vi "Get Exp Time.vi"(0 "Notifier Name":string, 11 "Error In":errorcluster) -> (4 "Notifier Name DUP":string, 8 "Exp Time (s)":dbl, 15 "Error Out":errorcluster)   [LabVIEW 2020]
uses:
  Hardware Configuration/Hardware Configuration Controls/Company.ctl
  Hamamatsu/Orca Flash/Orca Flash Controls/Orca Flash Parameters.ctl
  Hamamatsu/Orca Flash/Orca Flash Controls/Orca Flash Parameter List.ctl
  Hamamatsu/Orca Flash/Orca Flash Controls/Orca Flash Actions.ctl
  IDS/IDS Controls/IDS Actions.ctl
  IDS/IDS Controls/IDS Parameters.ctl
  IDS/IDS Controls/IDS Parameter List.ctl
  Photometrics/Prime BSI/R Cubed SITK/Prime BSI R3 Controls/Prime R3 Actions.ctl
  Photometrics/Prime BSI/R Cubed SITK/Prime BSI R3 Controls/Prime R3 Parameters.ctl
  Photometrics/Prime BSI/R Cubed SITK/Prime BSI R3 Controls/Prime R3 Parameter List.ctl
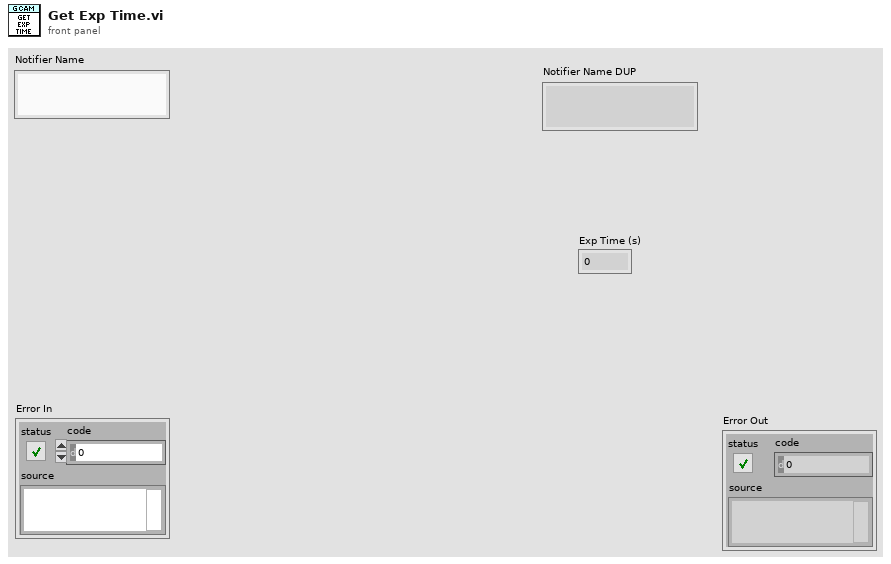
[diagram p1: front panel]
types:
  T1 = typedef "Company.ctl" = enum16{"AA Opto Electronic", "ASI", "Coherent", "Creset Optics", "CVI", "DAQmx", "Hamamatsu", "IDS", "Mad City Labs", "Marzhauser", "Measurement Computing", "MPB Com", "Olympus", "Photometrics", "PI", "Prior", "Thorlabs"}
  T2 = typedef "Orca Flash Actions.ctl" = enum16{"Idle", "Preview", "Record", "Record Settings", "Set Param", "Get Param", "Set ROI", "Get ROI", "Trigger Source", "Trigger Type", "Progessive Mode", "Area Mode", "Status", "Quit"}
  T3 = typedef "Orca Flash Parameters.ctl" = cluster{"Value":dbl, "Parameter":T4}
  T4 = typedef "Orca Flash Parameter List.ctl" = u32
  T5 = typedef "IDS Parameter List.ctl" = enum16{"Exposure Time (s)", "Binning"}
  T6 = typedef "IDS Parameters.ctl" = cluster{"Parameter":T5, "Value":dbl}
  T7 = typedef "IDS Actions.ctl" = enum16{"Error Check", "Initialize", "Preview", "Record", "Abort", "Record Settings", "Set Parameter", "Get Parameter", "Set ROI", "Get ROI", "Status", "Quit"}
  T8 = typedef "Prime R3 Parameter List.ctl" = enum16{"Exposure Time (s)"}
  T9 = typedef "Prime R3 Parameters.ctl" = cluster{"Parameter":T8, "Value":dbl}
  T10 = typedef "Prime R3 Actions.ctl" = enum16{"Error Check", "Initialize", "Preview", "Record", "Abort", "Record Settings", "Set Parameter", "Get Parameter", "Set ROI", "Get ROI", "Status", "Set Trigger", "Quit"}
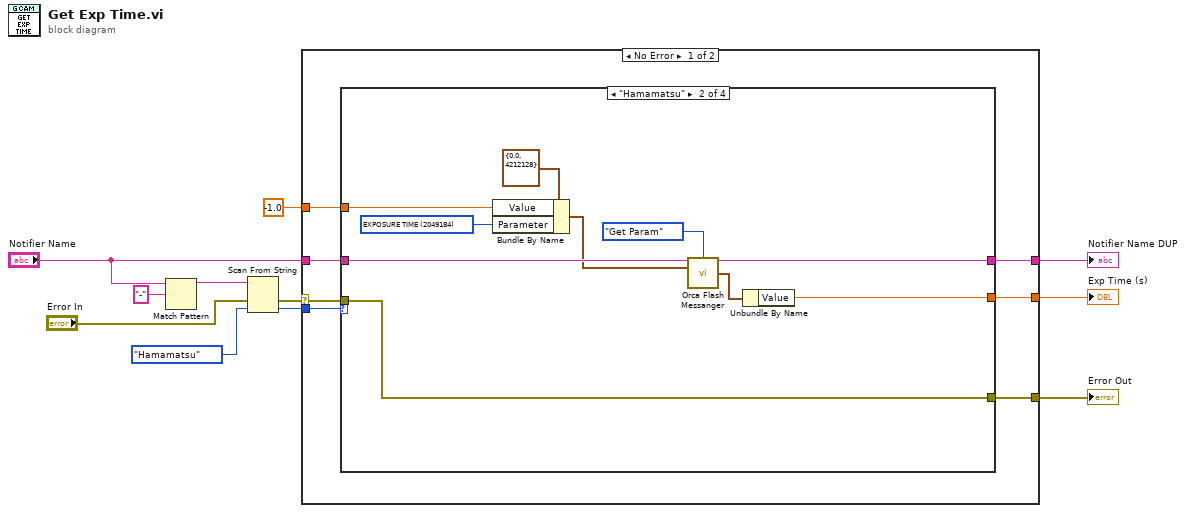
[diagram p0: block diagram]
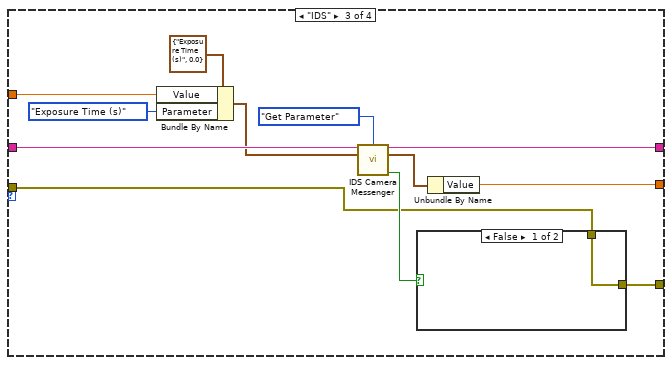
[diagram p3: hidden frame]
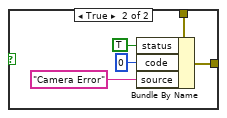
[diagram p4: hidden frame]
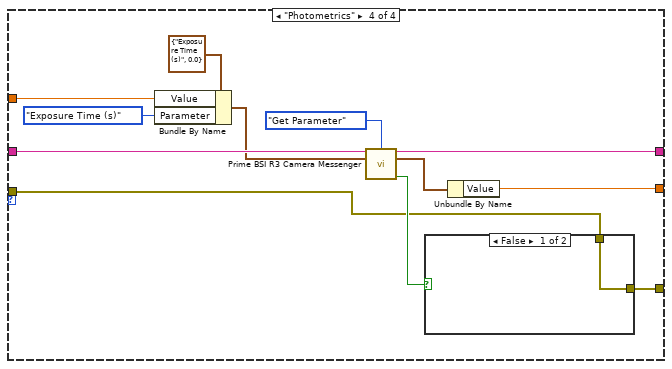
[diagram p5: hidden frame]
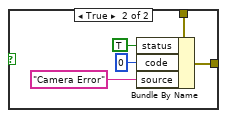
[diagram p6: hidden frame]
diagram:
  n1 = Match Pattern(string="Notifier Name", regular expression="-") -> (before substring=w9:string)  [unwired: 1 in, 3 out]
  n2 = Scan From String(input string=w9, error in="Error In", default 1=Company."Hamamatsu" ("Company")) -> (error out=w5:errorcluster, output 1=w8:T1)  [unwired: 2 in, 2 out]
  n3 = case shown="No Error" w5 {
    selector: w5 -> [w16 w69]
    tunnel: w8 -> [w18 _]
    tunnel: "Notifier Name" -> [w17 w70]
    tunnel: [w15 w70] -> w4
    tunnel: [w14 w69] -> w3
    tunnel: -1.0 -> [w13 w68]
    tunnel: [w12 w68] -> w1
    frame No Error {
      n4 = case shown="\"Hamamatsu\"" w18 {
        tunnel: w17 -> [w21 w31 w43 w61]
        tunnel: w16 -> [w20 w29 w39 w58]
        tunnel: [w21 w30 w42 w60] -> w15
        tunnel: [w20 w29 w38 w57] -> w14
        tunnel: w13 -> [w19 w26 w36 w54]
        tunnel: [w19 w23 w32 w50] -> w12
        frame Default {
        }
        frame "Hamamatsu" {
          w28 = T4 2049184 items=["SENSOR MODE"=4212128, "READOUT SPEED"=4211872, "READOUT DIRECTION"=4211904, "TRIGGER GLOBAL EXPOSURE"=2049680, "TRIGGER DELAY"=1066480, "SYNC READOUT SYSTEM BLANK"=1066528, "SENSOR COOLER"=2115248, "SENSOR COOLER STATUS"=2115280, "EXPOSURE TIME"=2049184, "DEFECT CORRECT MODE"=4670368, "BINNING"=4215968, "INTERNAL LINE SPEED"=4226000, "INTERNAL LINE INTERVAL"=4226016, "IMAGE PIXEL TYPE"=4343296, "NUMBER OF OUTPUT TRIGGER CONNECTOR"=1852320, "OUTPUT TRIGGER SOURCE[0]"=1852576, "OUTPUT TRIGGER SOURCE[1]"=1852832, "OUTPUT TRIGGER SOURCE[2]"=1853088, "OUTPUT TRIGGER POLARITY[0]"=1852592, "OUTPUT TRIGGER POLARITY[1]"=1852848, "OUTPUT TRIGGER POLARITY[2]"=1853104, "OUTPUT TRIGGER ACTIVE[0]"=1852608, "OUTPUT TRIGGER ACTIVE[1]"=1852864, "OUTPUT TRIGGER ACTIVE[2]"=1853120, "OUTPUT TRIGGER DELAY[0]"=1852624, "OUTPUT TRIGGER DELAY[1]"=1852880, "OUTPUT TRIGGER DELAY[2]"=1853136, "OUTPUT TRIGGER PERIOD[0]"=1852640, "OUTPUT TRIGGER PERIOD[1]"=1852896, "OUTPUT TRIGGER PERIOD[2]"=1853152, "OUTPUT TRIGGER KIND[0]"=1852656, "OUTPUT TRIGGER KIND[1]"=1852912, "OUTPUT TRIGGER KIND[2]"=1853168, "OUTPUT TRIGGER PRE HSYNC COUNT"=1852704] ("Parameter")
          n5 = Bundle By Name(cluster=T3 {"Value"=0.0, "Parameter"=4212128} ("sCMOS Parameter"), "Value"=w26, "Parameter"=w28) -> (w25:T3)
          n6 = call "Orca Flash Messanger.vi"("Notifier Name"=w31, "Camera Actions"=Orca_Flash_Actions."Get Param", "sCMOS Parameter"=w25) -> ("Notifier Name Dup"=w30:string, "sCMOS Parameter"=w24:T3)  [unwired: 8 in, 3 out]
          n7 = Unbundle By Name(w24) -> ("Value"=w23:dbl)
        }
        frame "IDS" {
          n8 = Bundle By Name(cluster=T6 {"Parameter"=enum."Exposure Time (s)", "Value"=0.0} ("IDS Parameter"), "Value"=w36, "Parameter"=IDS_Parameter_List."Exposure Time (s)") -> (w34:T6)
          n9 = call "IDS Camera Messenger.vi"("Notifier Name"=w43, "IDS Actions"=IDS_Actions."Get Parameter", "IDS Parameter"=w34) -> ("Notifier Name (Dup)"=w42:string, "IDS Parameter"=w33:T6, "Error?"=w40:bool)  [unwired: 7 in, 3 out]
          n10 = case shown="False" w40 {
            tunnel: w39 -> [w44 w49]
            tunnel: [w44 w48] -> w38
            frame False {
            }
            frame True {
              n11 = Bundle By Name(cluster=w49, "status"=TRUE, "code"=0, "source"="Camera Error") -> (w48:errorcluster)
            }
          }
          n12 = Unbundle By Name(w33) -> ("Value"=w32:dbl)
        }
        frame "Photometrics" {
          n13 = Bundle By Name(cluster=T9 {"Parameter"=enum."Exposure Time (s)", "Value"=0.0} ("Prime Parameter"), "Value"=w54, "Parameter"=Prime_R3_Parameter_List."Exposure Time (s)") -> (w52:T9)
          n14 = call "Prime BSI R3 Camera Messenger.vi"("Notifier Name"=w61, "Prime Actions"=Prime_R3_Actions."Get Parameter", "Prime Parameter"=w52) -> ("Notifier Name (Dup)"=w60:string, "Prime Parameter"=w51:T9, "Error?"=w59:bool)  [unwired: 7 in, 3 out]
          n15 = case shown="False" w59 {
            tunnel: w58 -> [w62 w67]
            tunnel: [w62 w66] -> w57
            frame False {
            }
            frame True {
              n16 = Bundle By Name(cluster=w67, "status"=TRUE, "code"=0, "source"="Camera Error") -> (w66:errorcluster)
            }
          }
          n17 = Unbundle By Name(w51) -> ("Value"=w50:dbl)
        }
      }
    }
    frame Error {
    }
  }
  "Error Out" <- w3
  "Notifier Name DUP" <- w4
  "Exp Time (s)" <- w1
